vi "niFPGA FFT Insert Bit Into Integer.vi"(0 "integer":u16, 5 "input value":bool, 7 "index":fxp<+,4,4>) -> (4 "output integer":u16)   [LabVIEW 2017]
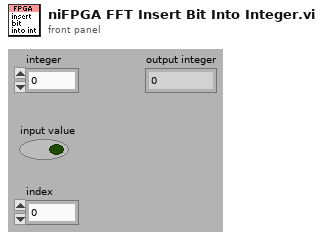
[diagram p1: front panel]
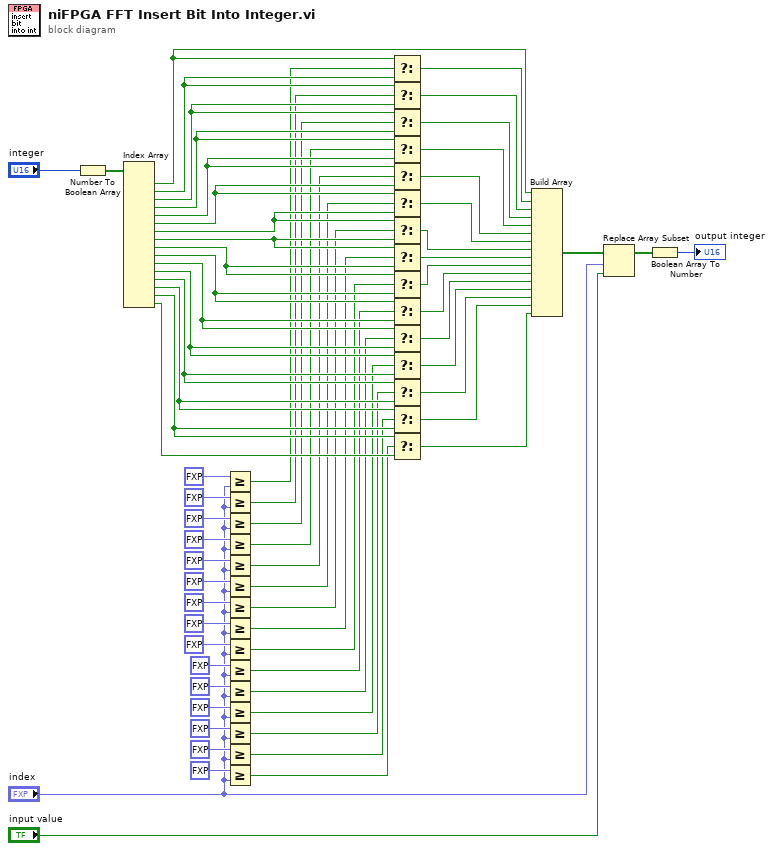
[diagram p0: block diagram]
diagram:
  n1 = Number To Boolean Array(number="integer") -> (Boolean array=w67:bool[])
  n2 = Index Array(array=w67) -> (element #1=w62:bool, element #2=w61:bool, element #3=w60:bool, element #4=w59:bool, element #5=w58:bool, element #6=w57:bool, element #7=w56:bool, element #8=w55:bool, element #9=w54:bool, element #10=w53:bool, element #11=w52:bool, element #12=w51:bool, element #13=w50:bool, element #14=w49:bool, element #15=w48:bool, element #16=w47:bool)  [unwired: 16 in]
  n3 = Greater Or Equal?(x=fxp<+,4,4> 1.0, y="index") -> (x >= y?=w16:bool)
  n4 = Greater Or Equal?(x=fxp<+,4,4> 2.0, y="index") -> (x >= y?=w15:bool)
  n5 = Greater Or Equal?(x=fxp<+,4,4> 3.0, y="index") -> (x >= y?=w14:bool)
  n6 = Greater Or Equal?(x=fxp<+,4,4> 4.0, y="index") -> (x >= y?=w13:bool)
  n7 = Greater Or Equal?(x=fxp<+,4,4> 5.0, y="index") -> (x >= y?=w12:bool)
  n8 = Greater Or Equal?(x=fxp<+,4,4> 6.0, y="index") -> (x >= y?=w11:bool)
  n9 = Greater Or Equal?(x=fxp<+,4,4> 7.0, y="index") -> (x >= y?=w10:bool)
  n10 = Greater Or Equal?(x=fxp<+,4,4> 8.0, y="index") -> (x >= y?=w9:bool)
  n11 = Greater Or Equal?(x=fxp<+,4,4> 9.0, y="index") -> (x >= y?=w8:bool)
  n12 = Greater Or Equal?(x=fxp<+,4,4> 10.0, y="index") -> (x >= y?=w7:bool)
  n13 = Greater Or Equal?(x=fxp<+,4,4> 11.0, y="index") -> (x >= y?=w6:bool)
  n14 = Greater Or Equal?(x=fxp<+,4,4> 12.0, y="index") -> (x >= y?=w5:bool)
  n15 = Greater Or Equal?(x=fxp<+,4,4> 13.0, y="index") -> (x >= y?=w4:bool)
  n16 = Greater Or Equal?(x=fxp<+,4,4> 14.0, y="index") -> (x >= y?=w3:bool)
  n17 = Greater Or Equal?(x=fxp<+,4,4> 15.0, y="index") -> (x >= y?=w2:bool)
  n18 = Select(t=w62, s=w16, f=w61) -> (s? t:f=w63:bool)
  n19 = Select(t=w61, s=w15, f=w60) -> (s? t:f=w46:bool)
  n20 = Select(t=w60, s=w14, f=w59) -> (s? t:f=w45:bool)
  n21 = Select(t=w59, s=w13, f=w58) -> (s? t:f=w44:bool)
  n22 = Select(t=w58, s=w12, f=w57) -> (s? t:f=w43:bool)
  n23 = Select(t=w57, s=w11, f=w56) -> (s? t:f=w42:bool)
  n24 = Select(t=w56, s=w10, f=w55) -> (s? t:f=w41:bool)
  n25 = Select(t=w55, s=w9, f=w54) -> (s? t:f=w40:bool)
  n26 = Select(t=w54, s=w8, f=w53) -> (s? t:f=w39:bool)
  n27 = Select(t=w53, s=w7, f=w52) -> (s? t:f=w38:bool)
  n28 = Select(t=w52, s=w6, f=w51) -> (s? t:f=w37:bool)
  n29 = Select(t=w51, s=w5, f=w50) -> (s? t:f=w36:bool)
  n30 = Select(t=w50, s=w4, f=w49) -> (s? t:f=w35:bool)
  n31 = Select(t=w49, s=w3, f=w48) -> (s? t:f=w34:bool)
  n32 = Select(t=w48, s=w2, f=w47) -> (s? t:f=w33:bool)
  n33 = Build Array(w62, w63, w46, w45, w44, w43, w42, w41, w40, w39, w38, w37, w36, w35, w34, w33) -> (w64:bool[])
  n34 = Replace Array Subset(array=w64, new element="input value", index="index") -> (w66:bool[])
  n35 = Boolean Array To Number(Boolean array=w66) -> (number=→"output integer":u16)
